vi "Add Log File.vi"(8 "error in (no error)":errorcluster, 11 "Node Ptr":T1=18446744073709551615 format="%.0x") -> (0 "error out":errorcluster, 3 "Node Ptr out":T1 format="%.0x")   [LabVIEW 2019, in "Telemetry System Explorer.lvlib"]
uses:
  Telemetry System Explorer.lvlib
  <vilib>/NI VeriStand/Custom Device API/Custom Device Item Ref.ctl
  <vilib>/NI VeriStand/Custom Device API/Custom Device API.lvlib
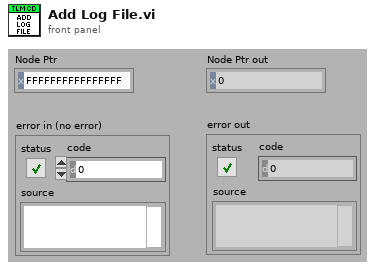
[diagram p1: front panel]
types:
  T1 = typedef "Custom Device API.lvlib/Custom Device Item Ref.ctl" = u64
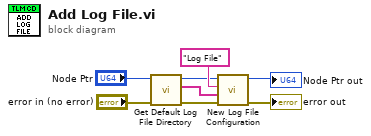
[diagram p0: block diagram]
diagram:
  n1 = call "Get Default Log File Directory.vi"("error in"="error in (no error)", "Device Item Ref In"="Node Ptr") -> ("error out"=w3:errorcluster, "Log File Directory String Array"=w6:string[], "Device Item Ref Out"=w2:T1)  [unwired: 7 in]
  n2 = call "New Log File Configuration.vi"("error in (no error)"=w3, "Default Log Directory"=w6, "Default Name"="Log File", "Device Ref in"=w2) -> ("error out"=→"error out":errorcluster, "Device Ref out"=→"Node Ptr out":T1)  [unwired: 6 in]
